vi "Log Data DBL.vi"(7 "Time Stamp":timestamp format="%<%x %.3X>T", 8 "error in":errorcluster, 9 "DBL":dbl, 10 "Ident":string, 11 "ISeries Actor in":refnum<class "ISeries Actor.lvclass">) -> (0 "error out":errorcluster, 3 "ISeries Actor out":refnum<class "ISeries Actor.lvclass">)   [LabVIEW 2023, in "ISeries Actor.lvlib" / "ISeries Actor.lvclass"]
uses:
  ISeries Actor.lvclass
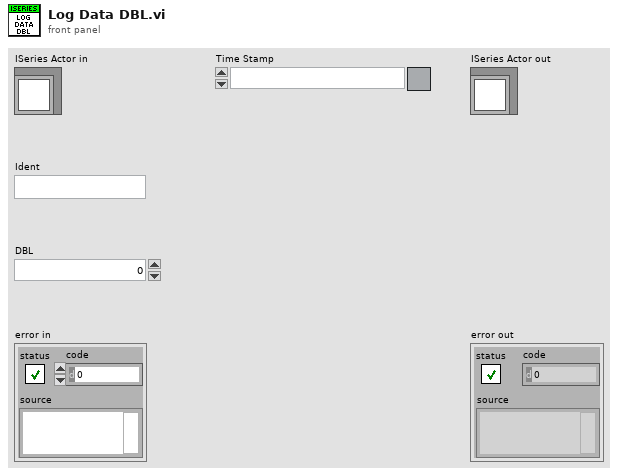
[diagram p1: front panel]
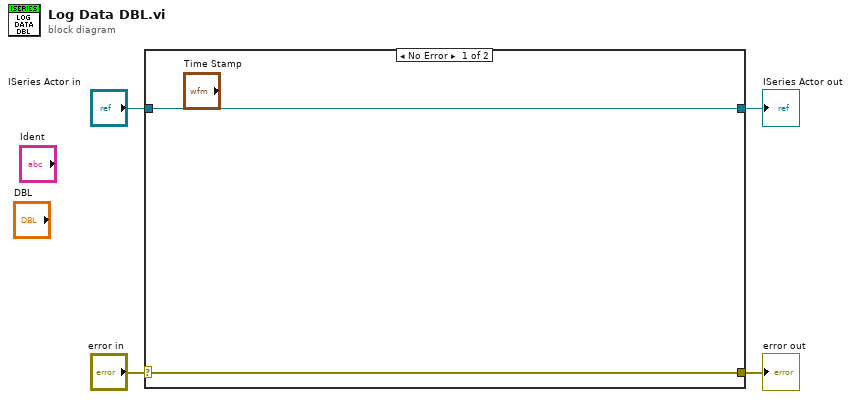
[diagram p0: block diagram]
diagram:
  n1 = case shown="No Error" "error in" {
    selector: "error in" -> [w5 w8]
    tunnel: [w5 w8] -> w3
    tunnel: [w6 w7] -> w1
    tunnel: "ISeries Actor in" -> [w6 w7]
    frame No Error {
    }
    frame Error {
    }
  }
  "error out" <- w3
  "ISeries Actor out" <- w1
